vi "Checksum.vi"(8 "error in":errorcluster, 10 "Command String":string="01K000004", 11 "VISA resource name":refnum<visa-resource-name>) -> (0 "error out":errorcluster, 1 "Checksum":string, 2 "Command String with Checksum":string, 3 "VISA resource name out":refnum<visa-resource-name>)   [LabVIEW 2010, in "FEM-03.lvlib"]
doc: "Performs checksum"
uses:
  FEM-03.lvlib
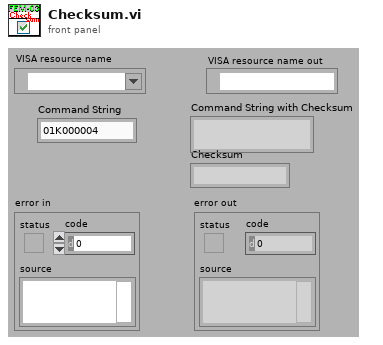
[diagram p1: front panel]
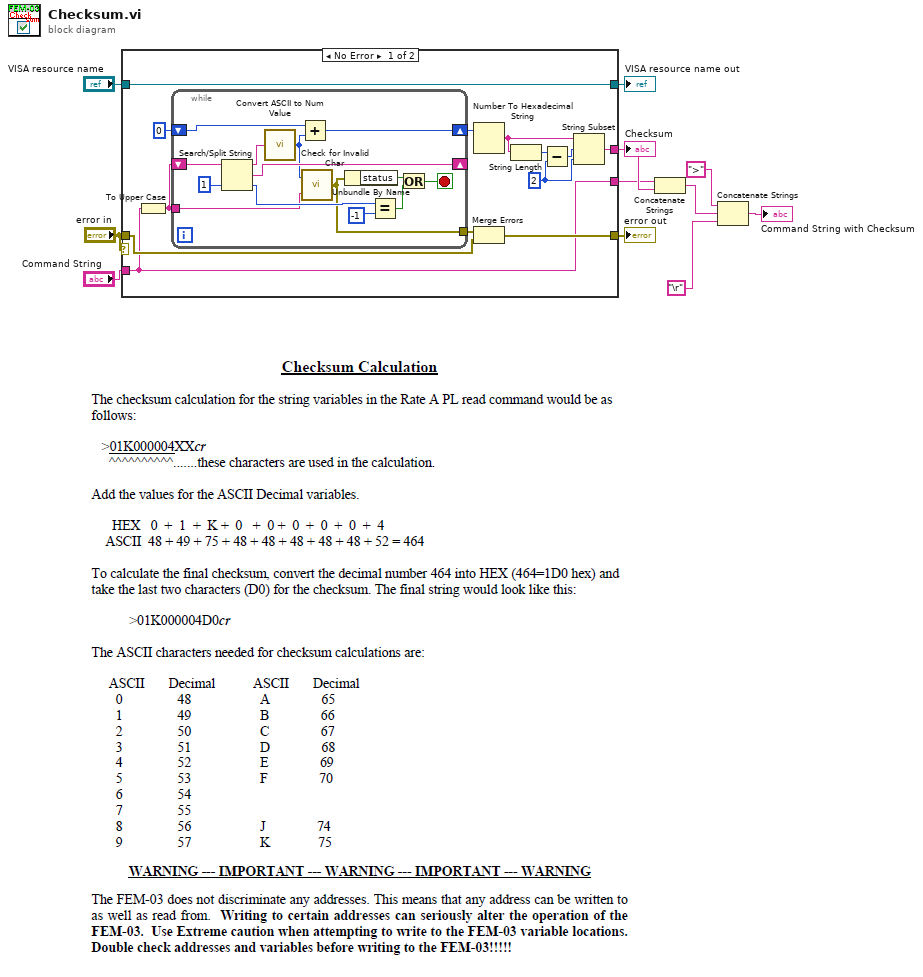
[diagram p0: block diagram]
diagram:
  n1 = case shown="No Error" "error in" {
    tunnel: "Command String" -> [w12 w39]
    tunnel: "VISA resource name" -> [w14 w40]
    tunnel: [w17 w41] -> w7
    tunnel: "error in" -> [w15 w41]
    tunnel: [w14 w40] -> w10
    tunnel: [w13 _] -> w6
    tunnel: [w12 w39] -> w5
    frame No Error {
      w21 = 2 ("length (rest)")
      n2 = To Upper Case(1:w12) -> (0:w18:string)
      n3 = while {
        shift-right: [w33] -> _
        shift-left: w18 -> [w38]
        shift-right: [w31] -> w19
        shift-left: 0 -> [w30]
        tunnel: w18 -> [w29]
        tunnel: [w26] -> w16
        stop <- w28 stop-if-true
        n4 = Search/Split String(string=w38, offset (0)=1) -> (substring before match=w32:string, match + rest of string=w33:string, offset of match=w36:i32)  [unwired: 1 in]
        n5 = call "Convert ASCII to Num Value.vi"("String"=w32) -> ("ASCII Num Value"=w25:i32)
        n6 = Add(x=w30, y=w25) -> (x+y=w31:i32)
        n7 = call "Check for Invalid Char.vi"("String"=w29, "ASCII Num Value"=w25) -> ("error out"=w26:errorcluster)
        n8 = Unbundle By Name(w26) -> ("status"=w27:bool)
        n9 = Equal?(x=w36, y=-1) -> (x = y?=w34:bool)
        n10 = Or(x=w27, y=w34) -> (x .or. y?=w28:bool)
      }
      n11 = Number To Hexadecimal String(2:w19) -> (0:w23:string)  [unwired: 1 in]
      n12 = Merge Errors(w16, w15) -> (w17:errorcluster)
      n13 = String Length(string=w23) -> (length=w20:i32)
      n14 = Subtract(x=w20, y=w21) -> (x-y=w22:i32)
      n15 = String Subset(string=w23, offset (0)=w22, length (rest)=w21) -> (substring=w13:string)
    }
    frame Error {
    }
  }
  "VISA resource name out" <- w10
  "error out" <- w7
  "Checksum" <- w6
  n16 = Concatenate Strings(w5, w6) -> (w3:string)
  n17 = Concatenate Strings(">" ("string"), w3, "\r") -> (→"Command String with Checksum":string)
